vi "FTW-JSON-LexicalScan-Parse.vi"(0 "JSON String":T1, 11 "error in":errorcluster) -> (4 "JSON String Out":T1, 6 "Name":string, 8 "Container":variant, 15 "error out":errorcluster)   [LabVIEW 2015]
uses:
  FTW-JSON-LexicalScan.ctl
panel:
  # "Inputs"
  # "Outputs"
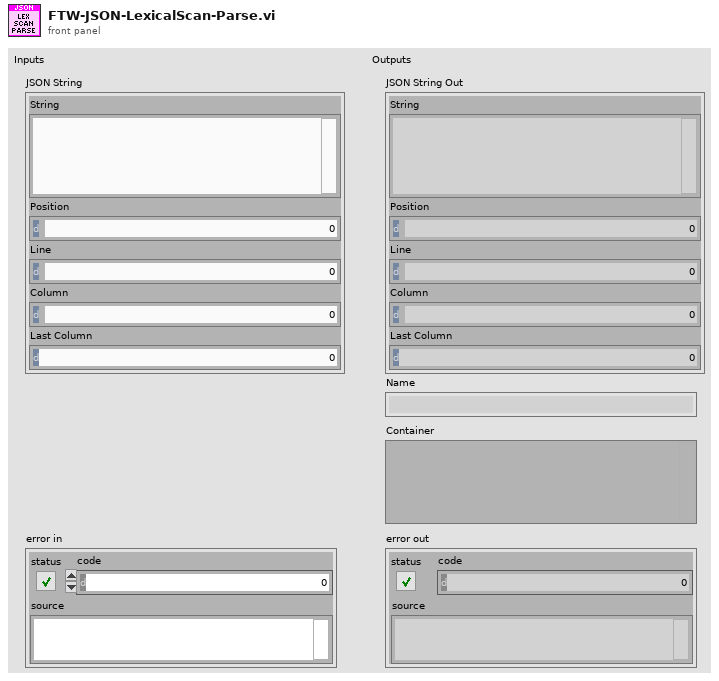
[diagram p1: front panel]
types:
  T1 = typedef "FTW-JSON-LexicalScan.ctl" = cluster{"String":string, "Position":i32, "Line":i32, "Column":i32, "Last Column":i32}
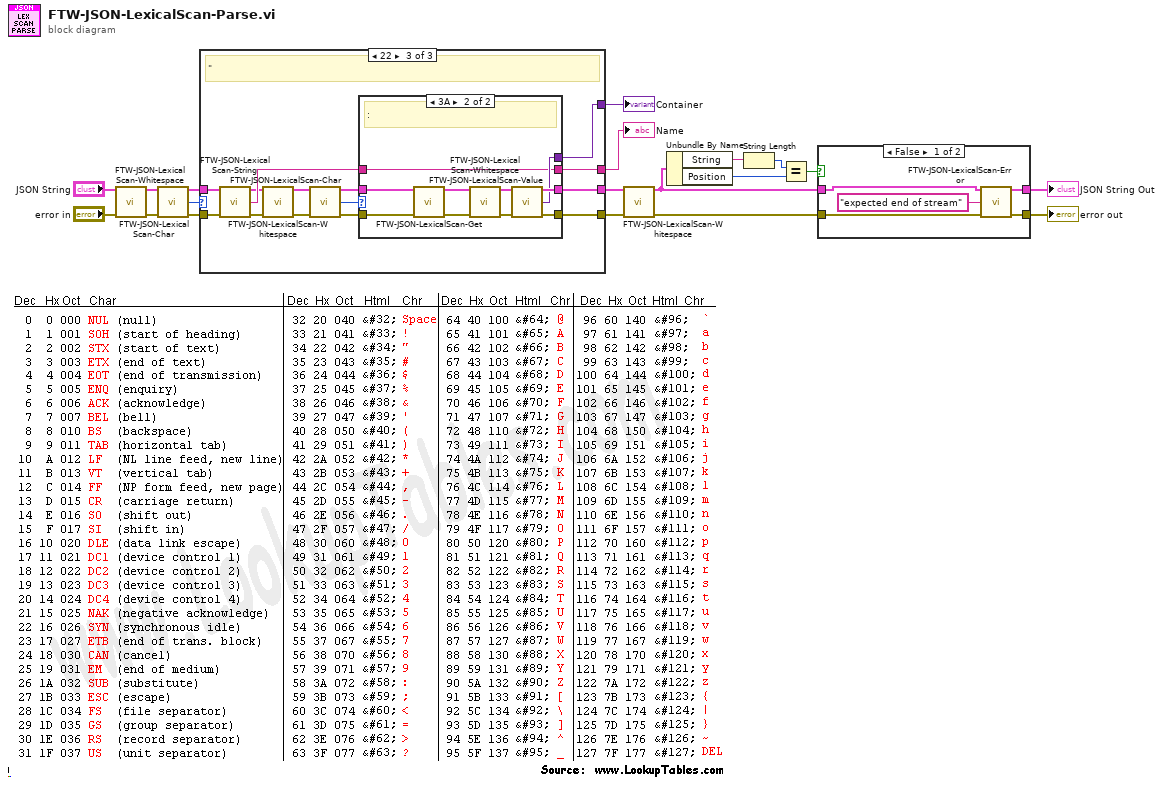
[diagram p0: block diagram]
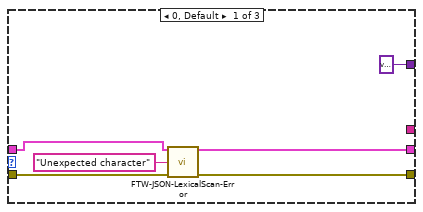
[diagram p3: hidden frame]
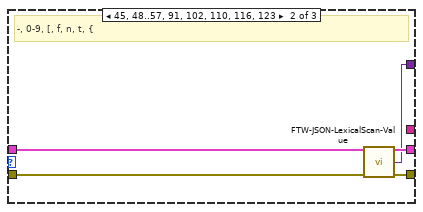
[diagram p4: hidden frame]
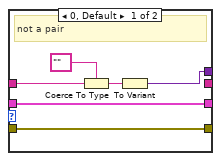
[diagram p5: hidden frame]
diagram:
  n1 = call "FTW-JSON-LexicalScan-Whitespace.vi"("JSON String"="JSON String", "error in"="error in") -> ("JSON String Out"=w11:T1, "error out"=w13:errorcluster)  [unwired: 12 in]
  n2 = call "FTW-JSON-LexicalScan-Char.vi"("JSON String"=w11, "error in"=w13) -> ("JSON String Out"=w16:T1, "Char"=w18:u8, "error out"=w17:errorcluster)  [unwired: 11 in]
  n3 = case shown="22" w18 {
    tunnel: w17 -> [w25 w29 w43]
    tunnel: w16 -> [w22 w30 w44]
    tunnel: [w23 w28 w37] -> w15
    tunnel: [w21 w27 w38] -> w8
    tunnel: [variant w26 w32] -> w14
    tunnel: [_ _ w31] -> w10
    frame 0, Default {
      n4 = call "FTW-JSON-LexicalScan-Error.vi"("JSON String"=w22, "Error String"="Unexpected character", "error in"=w25) -> ("JSON String Out"=w21:T1, "error out"=w23:errorcluster)  [unwired: 11 in]
    }
    frame 45, 48..57, 91, 102, 110, 116, 123 {
      # "-, 0-9, [, f, n, t, {"
      n5 = call "FTW-JSON-LexicalScan-Value.vi"("JSON String"=w30, "error in"=w29) -> ("JSON String Out"=w27:T1, "Container"=w26:variant, "error out"=w28:errorcluster)  [unwired: 11 in]
    }
    frame 34 {
      # "\""
      n6 = call "FTW-JSON-LexicalScan-String.vi"("JSON String"=w44, "error in"=w43) -> ("JSON String Out"=w34:T1, "String"=w36:string, "error out"=w42:errorcluster)  [unwired: 11 in]
      n7 = call "FTW-JSON-LexicalScan-Whitespace.vi"("JSON String"=w34, "error in"=w42) -> ("JSON String Out"=w33:T1, "error out"=w35:errorcluster)  [unwired: 12 in]
      n8 = call "FTW-JSON-LexicalScan-Char.vi"("JSON String"=w33, "error in"=w35) -> ("JSON String Out"=w40:T1, "Char"=w41:u8, "error out"=w39:errorcluster)  [unwired: 11 in]
      n9 = case shown="3A" w41 {
        tunnel: w39 -> [w50 w60]
        tunnel: [w50 w55] -> w37
        tunnel: w40 -> [w49 w57]
        tunnel: [w49 w53] -> w38
        tunnel: [w47 w52] -> w32
        tunnel: w36 -> [w48 w51]
        tunnel: [_ w51] -> w31
        frame 0, Default {
          # "not a pair"
          n10 = Coerce To Type(0:w48, 1:"") -> (2:w46:string)
          n11 = To Variant(anything=w46) -> (Variant=w47:variant)
        }
        frame 58 {
          # ":"
          n12 = call "FTW-JSON-LexicalScan-Get.vi"("JSON String"=w57, "error in"=w60) -> ("JSON String Out"=w56:T1, "error out"=w58:errorcluster)  [unwired: 11 in, 1 out]
          n13 = call "FTW-JSON-LexicalScan-Whitespace.vi"("JSON String"=w56, "error in"=w58) -> ("JSON String Out"=w54:T1, "error out"=w59:errorcluster)  [unwired: 12 in]
          n14 = call "FTW-JSON-LexicalScan-Value.vi"("JSON String"=w54, "error in"=w59) -> ("JSON String Out"=w53:T1, "Container"=w52:variant, "error out"=w55:errorcluster)  [unwired: 11 in]
        }
      }
    }
  }
  "Container" <- w14
  "Name" <- w10
  n15 = call "FTW-JSON-LexicalScan-Whitespace.vi"("JSON String"=w8, "error in"=w15) -> ("JSON String Out"=w2:T1, "error out"=w9:errorcluster)  [unwired: 12 in]
  n16 = Unbundle By Name(w2) -> ("String"=w7:string, "Position"=w5:i32)
  n17 = String Length(string=w7) -> (length=w6:i32)
  n18 = Equal?(x=w6, y=w5) -> (x = y?=w1:bool)
  n19 = case shown="False" w1 {
    tunnel: w9 -> [w65 w66]
    tunnel: [w64 w66] -> w4
    tunnel: [w63 w67] -> w3
    tunnel: w2 -> [w62 w67]
    frame False {
      n20 = call "FTW-JSON-LexicalScan-Error.vi"("JSON String"=w62, "Error String"="expected end of stream", "error in"=w65) -> ("JSON String Out"=w63:T1, "error out"=w64:errorcluster)  [unwired: 11 in]
    }
    frame True {
    }
  }
  "error out" <- w4
  "JSON String Out" <- w3
